vi "Get Frames.vi"(8 "error in":errorcluster, 11 "Incoming/Outgoing in":T1 format="%.0x") -> (0 "error out":errorcluster, 2 "Frames":T1[](array[typedef]) format="%.0x", 3 "Incoming/Outgoing out":T1 format="%.0x")   [LabVIEW 2020, in "Communication Bus Template Scripting.lvlib"]
uses:
  <vilib>/NI VeriStand/Custom Device API/Custom Device Item Ref.ctl
  Constants.vi
  Communication Bus Template Scripting.lvlib
  <vilib>/NI VeriStand/Custom Device Tools/Custom Device Utility Library/Custom Device Utility Library.lvlib
  <vilib>/NI VeriStand/Custom Device Tools/Custom Device Utility Library/NI VeriStand - Search for All Items by GUID.vi
  <vilib>/NI VeriStand/Custom Device API/Custom Device API.lvlib
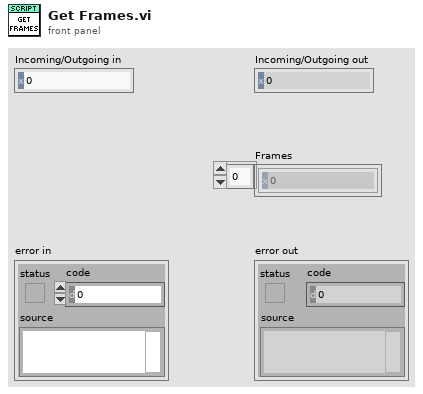
[diagram p1: front panel]
types:
  T1 = typedef "Custom Device API.lvlib/Custom Device Item Ref.ctl" = u64
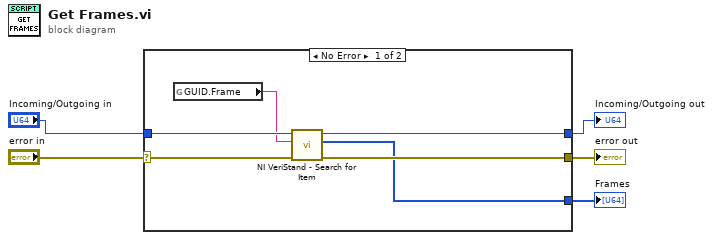
[diagram p0: block diagram]
diagram:
  n1 = case shown="No Error" "error in" {
    selector: "error in" -> [w9 w13]
    tunnel: "Incoming/Outgoing in" -> [w11 w12]
    tunnel: [w8 w13] -> w4
    tunnel: [w10 w12] -> w3
    tunnel: [w6 _] -> w1
    frame No Error {
      n2 = global read "Constants.vi" "GUID.Frame"() -> (w7:string)
      n3 = call-poly <vilib>:"NI VeriStand - Search for Item.vi"("error in"=w9, "Item GUID"=w7, "Section Ref in"=w11) -> ("error out"=w8:errorcluster, "Item Refs"=w6:T1[], "Section Ref out"=w10:T1)  [unwired: 5 in, 1 out]
    }
    frame Error {
    }
  }
  "error out" <- w4
  "Incoming/Outgoing out" <- w3
  "Frames" <- w1
